vi "GetType.vi"(8 "error in (no error)":errorcluster, 11 "Configure Start Trigger [STT] Msg":refnum<class "Configure Start Trigger [STT] Msg.lvclass">) -> (0 "error out":errorcluster, 2 "Data Sample":variant, 3 "Configure Start Trigger [STT] Msg":refnum<class "Configure Start Trigger [STT] Msg.lvclass">)   [LabVIEW 2015, in "CS++Fgen.lvlib" / "Configure Start Trigger [STT] Msg.lvclass"]
doc: "This VI delivers a sample of the data type format the message expects."
uses:
  Configure Start Trigger [STT] Msg.lvclass
  Configure Start Trigger [STT] Msg.lvclass/Configure Start Trigger [STT] Msg.ctl
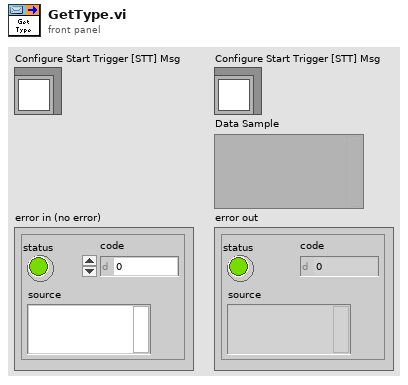
[diagram p1: front panel]
types:
  T1 = cluster{"Channel Name (\"\")":string, "Trigger Source (None)":string, "Trigger Slope (Positive)":i32}
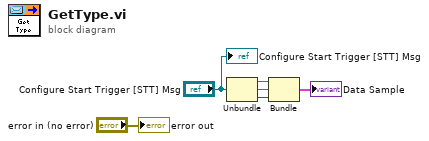
[diagram p0: block diagram]
diagram:
  n1 = Unbundle("Configure Start Trigger [STT] Msg") -> (w3:string, w2:string, w1:i32)
  n2 = Bundle("Channel Name (\"\")"=w3, "Trigger Source (None)"=w2, "Trigger Slope (Positive)"=w1) -> (→"Data Sample":T1)  [unwired: 1 in]
  "error out" <- "error in (no error)"
  "Configure Start Trigger [STT] Msg" <- "Configure Start Trigger [STT] Msg"
